vi "Fetch (Scaled and Reduced Resolution).vi"(0 "VISA resource name":refnum<visa-resource-name>, 1 "Segment Index (0)":i32 format="%.0g", 5 "Measurement Source (1: Channel 1)":i32(ring)=1 items=["Channel 1"=1, "Channel 2"=2, "Channel 3"=3, "Channel 4"=4, "Function 1"=5, "Function 2"=6, "Function 3"=7, "Function 4"=8, "Memory 1"=9, "Memory 2"=10, "Memory 3"=11, "Memory 4"=12], 7 "Waveform Size (0)":i32=1000 caption="Waveform Size (1000)", 9 "Maximum Time (10000ms)":u32=10000, 11 "error in (no error)":errorcluster) -> (4 "VISA resource name out":refnum<visa-resource-name>, 6 "Waveform Information":T1, 8 "Waveform Data":waveform(dbl)(graph), 15 "error out":errorcluster)   [LabVIEW 2013, in "Agilent 90000 Series.lvlib"]
doc: "Fetches a decimated and scaled waveform. If the instrument can perform the decimation before pass it to desktop, a decimated waveform will be read directly from the instrument and returned. Else all waveform points will be read from instrument in chunks and a decimation will be perform in the memory of desktop PC. This VI adopts Min/Max decimating method."
uses:
  Agilent 90000 Series.lvlib
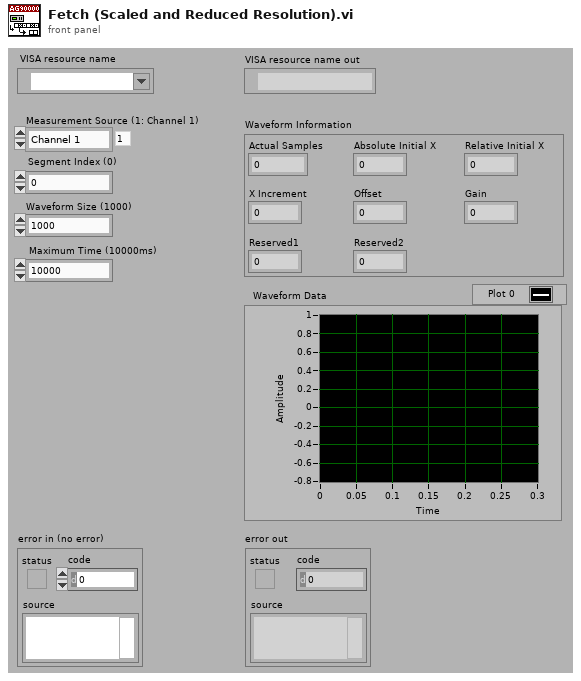
[diagram p1: front panel]
types:
  T1 = cluster{"Actual Samples":i32, "Absolute Initial X":dbl, "Relative Initial X":dbl, "X Increment":dbl, "Offset":dbl, "Gain":dbl, "Reserved1":dbl, "Reserved2":dbl}
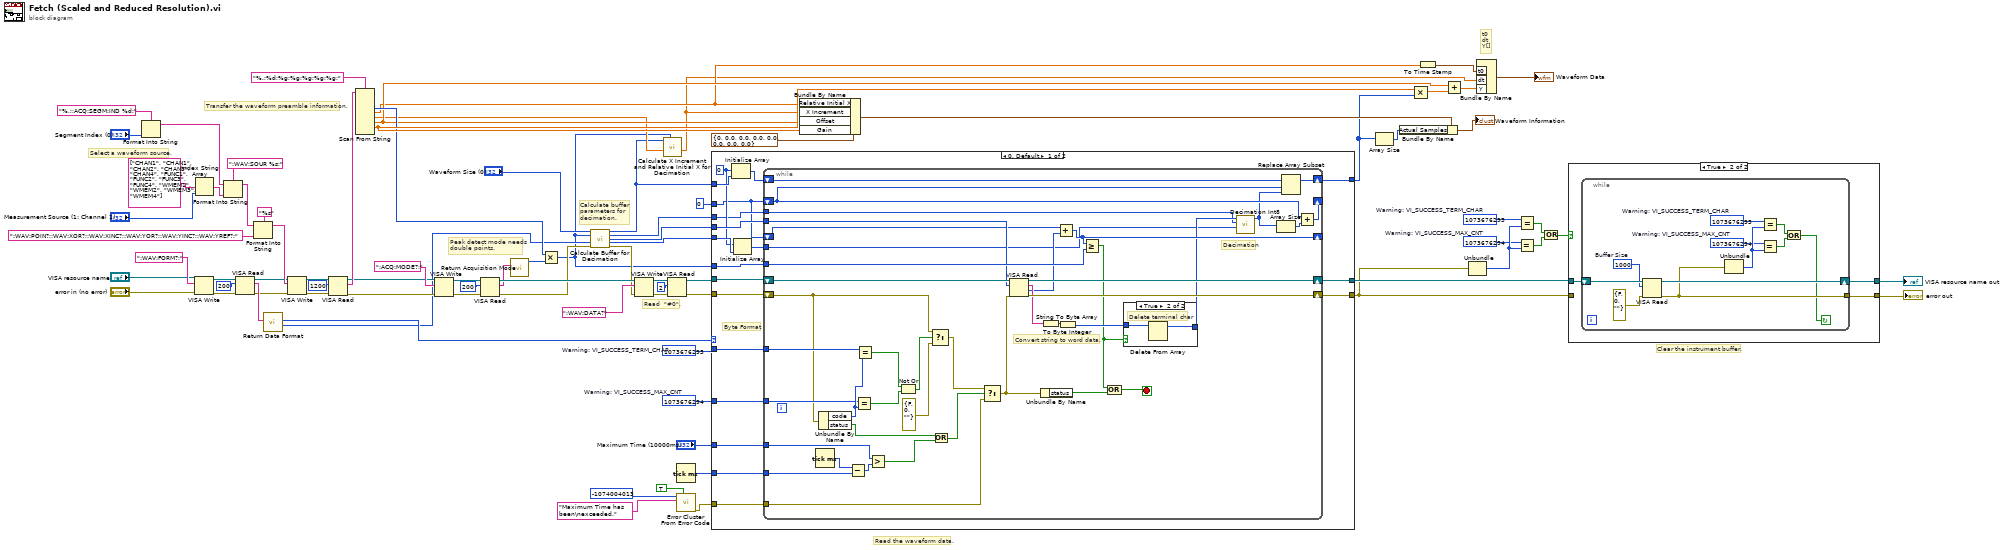
[diagram p0: block diagram]
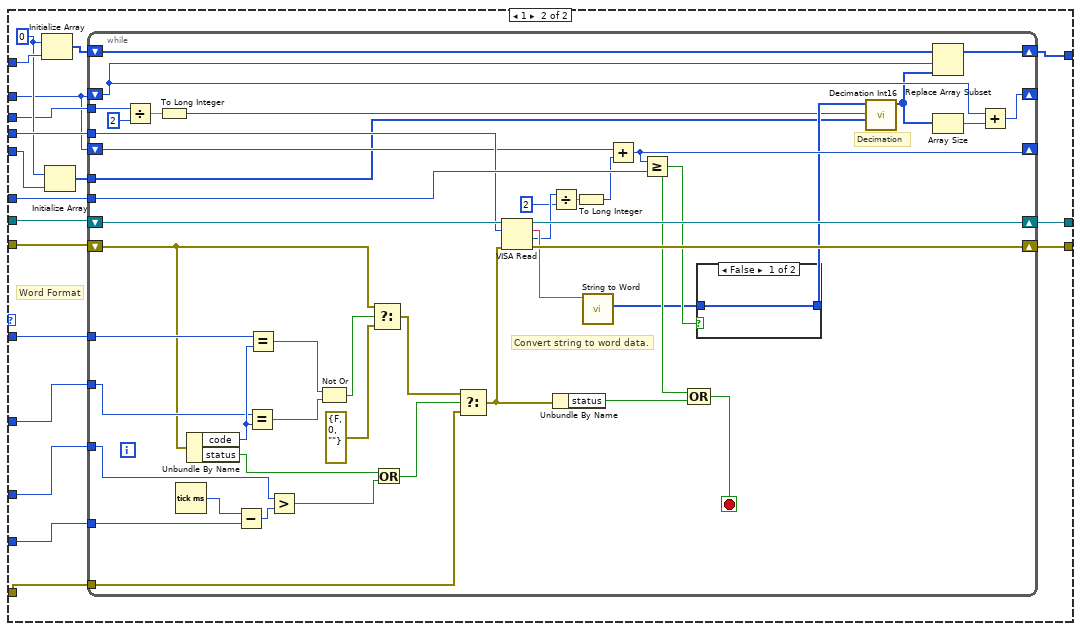
[diagram p3: hidden frame]
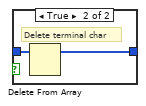
[diagram p4: hidden frame]
diagram:
  w50 = 1073676294  # Warning: VI_SUCCESS_MAX_CNT
  w51 = 1073676293  # Warning: VI_SUCCESS_TERM_CHAR
  w68 = 1073676294  # Warning: VI_SUCCESS_MAX_CNT
  w67 = 1073676293  # Warning: VI_SUCCESS_TERM_CHAR
  # "Calculate buffer \nparameters for \ndecimation."
  # "Read the waveform data."
  # "Peak detect mode needs\ndouble points."
  # "Read  \"#0\"."
  # "Select a waveform source."
  # "t0\ndt\nY[]"
  # "Clear the instrument buffer."
  # "Transfer the waveform preamble information."
  n1 = Format Into String(format string="%.;:ACQ:SEGM:IND %d;", "Segment Index (0)") -> (resulting string=w1:string)  [unwired: 2 in, 1 out]
  n2 = VISA Write(VISA resource name="VISA resource name", write buffer=":WAV:FORM?;", error in (no error)="error in (no error)") -> (VISA resource name out=w43:refnum<visa-resource-name>, error out=w42:errorcluster)  [unwired: 1 out]
  n3 = Index String Array(1:"Measurement Source (1: Channel 1)", 2:string[] ["CHAN1", "CHAN1", "CHAN2", "CHAN3", "CHAN4", "FUNC1", "FUNC2", "FUNC3", "FUNC4", "WMEM1", "WMEM2", "WMEM3", "WMEM4"] ("subarray 2")) -> (0:w76:string)  [unwired: 1 out]
  n4 = Format Into String(format string=":WAV:SOUR %s;" ("Source Command"), initial string=w1, w76) -> (resulting string=w79:string)  [unwired: 1 in, 1 out]
  n5 = VISA Read(VISA resource name=w43, byte count=u32 200, error in (no error)=w42) -> (VISA resource name out=w37:refnum<visa-resource-name>, read buffer=w34:string, error out=w11:errorcluster)  [unwired: 1 out]
  n6 = Format Into String(format string="%s", initial string=w79, ":WAV:POIN?;:WAV:XOR?;:WAV:XINC?;:WAV:YOR?;:WAV:YINC?;:WAV:YREF?;") -> (resulting string=w78:string)  [unwired: 1 in, 1 out]
  n7 = call "Return Data Format.vi"("String In"=w34) -> ("Bytes of Each Point"=w8:u8, "Data Format"=w25:u16)  [unwired: 1 in, 8 out]
  n8 = VISA Write(VISA resource name=w37, write buffer=w78, error in (no error)=w11) -> (VISA resource name out=w84:refnum<visa-resource-name>, error out=w83:errorcluster)  [unwired: 1 out]
  n9 = VISA Read(VISA resource name=w84, byte count=u32 1200, error in (no error)=w83) -> (VISA resource name out=w32:refnum<visa-resource-name>, read buffer=w62:string, error out=w12:errorcluster)  [unwired: 1 out]
  n10 = Scan From String(format string="%.;%d;%g;%g;%g;%g;%g;", input string=w62) -> (output 1=w28:i32, output 2=w13:dbl, output 3=w10:dbl, output 4=w14:dbl, output 5=w29:dbl)  [unwired: 2 in, 10 out]
  n11 = VISA Write(VISA resource name=w32, write buffer=":ACQ:MODE?;", error in (no error)=w12) -> (VISA resource name out=w58:refnum<visa-resource-name>, error out=w59:errorcluster)  [unwired: 1 out]
  n12 = VISA Read(VISA resource name=w58, byte count=u32 200, error in (no error)=w59) -> (VISA resource name out=w57:refnum<visa-resource-name>, read buffer=w15:string, error out=w18:errorcluster)  [unwired: 1 out]
  n13 = call "Return Acquisition Mode.vi"("Acquisition Mode"=w15) -> ("Multiply Factor"=w16:i32)  [unwired: 10 out]
  n14 = Multiply(x=w28, y=w16) -> (x*y=w6:i32)
  n15 = call "Calculate Buffer for Decimation.vi"("Waveform Size In (100)"="Waveform Size (0)", "Actual Points (1000)"=w6, "Bytes of Each Point (1)"=w8, "error in (no error)"=w18) -> ("Waveform Size Out"=w4:i32, "Number of Bytes per Chunck"=w5:i32, "Number of Bytes per Fetch"=w20:i32, "Decimation Buffer Size"=w19:i32, "error out"=w17:errorcluster)  [unwired: 7 out]
  n16 = VISA Write(VISA resource name=w57, write buffer=":WAV:DATA?" ("format string"), error in (no error)=w17) -> (VISA resource name out=w65:refnum<visa-resource-name>, error out=w64:errorcluster)  [unwired: 1 out]
  n17 = call "Calculate X Increment and Relative Initial X for Decimation.vi"("Actual Points (1000)"=w6, "Original X Increment (0)"=w10, "Waveform Size (100)"=w4) -> ("X Increment Out"=w9:dbl)  [unwired: 2 in, 6 out]
  n18 = VISA Read(VISA resource name=w65, byte count=u32 2, error in (no error)=w64) -> (VISA resource name out=w35:refnum<visa-resource-name>, error out=w36:errorcluster)  [unwired: 2 out]
  n19 = Tick Count (ms)() -> (millisecond timer value=w48:u32)
  n20 = call <vilib>:"Error Cluster From Error Code.vi"("show call chain? (False)"=TRUE, "error message (\"\")"="Maximum Time has been\nexceeded." ("error message (\"\")"), "error code (0)"=-1074004013) -> ("error out"=w45:errorcluster)  [unwired: 1 in, 5 out]
  n21 = case shown="0, Default" w25 {
    tunnel: [w103 w166] -> w74
    tunnel: [w102 w165] -> w73
    tunnel: w36 -> [w101 w164]
    tunnel: w35 -> [w100 w163]
    tunnel: [w99 w162] -> w23
    tunnel: w51 -> [w98 w161]
    tunnel: w50 -> [w97 w160]
    tunnel: "Maximum Time (10000ms)" -> [w96 w159]
    tunnel: w48 -> [w95 w158]
    tunnel: w45 -> [w94 w157]
    tunnel: w4 -> [w92 w155]
    tunnel: w20 -> [w91 w154]
    tunnel: w6 -> [w90 w153]
    tunnel: w19 -> [w89 w152]
    tunnel: w5 -> [w86 w149]
    tunnel: 0 ("index") -> [w85 w148]
    frame 0, Default {
      w88 = i8 0 ("element")
      # "Byte Format"
      n22 = Initialize Array(w88, w92) -> (w93:i8[])
      n23 = Initialize Array(w88, w89) -> (w87:i8[])
      n24 = while {
        shift-right: [w141] -> w102
        shift-left: w101 -> [w132]
        shift-right: [w144] -> w103
        shift-left: w100 -> [w143]
        shift-right: [w142] -> w99
        shift-left: w93 -> [w119]
        shift-right: [w140] -> _
        shift-left: w85 -> [w112]
        tunnel: w98 -> [w134]
        tunnel: w97 -> [w133]
        tunnel: w96 -> [w129]
        tunnel: w95 -> [w128]
        tunnel: w94 -> [w123]
        tunnel: w90 -> [w116]
        tunnel: w91 -> [w115]
        tunnel: w86 -> [w106]
        tunnel: w87 -> [w105]
        shift-right: [w110] -> _
        shift-left: w85 -> [w108]
        stop <- w120 stop-if-true
        # "Convert string to word data."
        # "Decimation"
        n25 = Tick Count (ms)() -> (millisecond timer value=w130:u32)
        n26 = Unbundle By Name(w132) -> ("code"=w135:i32, "status"=w127:bool)
        n27 = Subtract(x=w130, y=w128) -> (x-y=w131:u32)
        n28 = Equal?(x=w133, y=w135) -> (x = y?=w138:bool)
        n29 = Equal?(x=w134, y=w135) -> (x = y?=w139:bool)
        n30 = Greater?(x=w129, y=w131) -> (0:w126:bool)
        n31 = Not Or(1:w138, 2:w139) -> (0:w137:bool)
        n32 = Select(t=w132, s=w137, f=errorcluster {"status"=FALSE, "code"=0, "source"=""} ("error in (no error)")) -> (s? t:f=w125:errorcluster)
        n33 = Or(x=w127, y=w126) -> (x .or. y?=w124:bool)
        n34 = Select(t=w125, s=w124, f=w123) -> (s? t:f=w122:errorcluster)
        n35 = VISA Read(VISA resource name=w143, byte count=w115, error in (no error)=w122) -> (VISA resource name out=w144:refnum<visa-resource-name>, read buffer=w118:string, return count=w114:u32, error out=w141:errorcluster)
        n36 = Unbundle By Name(w122) -> ("status"=w121:bool)
        n37 = String To Byte Array(string=w118) -> (unsigned byte array=w117:u8[])
        n38 = Add(x=w112, y=w114) -> (x+y=w140:u32)
        n39 = To Byte Integer(number=w117) -> (8bit integer=w113:i8[])
        n40 = Greater Or Equal?(x=w140, y=w116) -> (x >= y?=w109:bool)
        n41 = Compound Arithmetic op=OR(w109, w121) -> (w120:bool)
        n42 = case shown="True" w109 {
          tunnel: w113 -> [w145 w147]
          tunnel: [w145 w146] -> w107
          frame False {
          }
          frame True {
            # "Delete terminal char"
            n43 = Delete From Array(array=w147) -> (array with subset deleted=w146:i8[])  [unwired: 2 in, 1 out]
          }
        }
        n44 = call "Decimation Int8.vi"("Decimation Array"=w105, "Number of Bytes per Chunck (1000)"=w106, "Raw Data"=w107) -> ("Decimation Data"=w104:i8[])  [unwired: 8 out]
        n45 = Array Size(array=w104) -> (size(s)=w111:i32)
        n46 = Replace Array Subset(array=w119, new element=w104, index=w108) -> (w142:i8[])
        n47 = Add(x=w108, y=w111) -> (x+y=w110:i32)
      }
    }
    frame 1 {
      w151 = i16 0 ("element")
      # "Word Format"
      n48 = Initialize Array(w151, w155) -> (w156:i16[])
      n49 = Initialize Array(w151, w152) -> (w150:i16[])
      n50 = while {
        shift-right: [w209] -> w165
        shift-left: w164 -> [w200]
        shift-right: [w212] -> w166
        shift-left: w163 -> [w211]
        shift-right: [w210] -> w162
        shift-left: w156 -> [w187]
        shift-right: [w208] -> _
        shift-left: w148 -> [w184]
        tunnel: w161 -> [w202]
        tunnel: w160 -> [w201]
        tunnel: w159 -> [w197]
        tunnel: w158 -> [w196]
        tunnel: w157 -> [w191]
        tunnel: w153 -> [w186]
        tunnel: w154 -> [w185]
        tunnel: w149 -> [w173]
        tunnel: w150 -> [w167]
        shift-right: [w181] -> _
        shift-left: w148 -> [w183]
        stop <- w188 stop-if-true
        # "Decimation"
        # "Convert string to word data."
        n51 = Divide(x=w173, y=2) -> (x/y=w172:dbl)
        n52 = To Long Integer(number=w172) -> (32bit integer=w168:i32)
        n53 = Tick Count (ms)() -> (millisecond timer value=w198:u32)
        n54 = Unbundle By Name(w200) -> ("code"=w203:i32, "status"=w195:bool)
        n55 = Subtract(x=w198, y=w196) -> (x-y=w199:u32)
        n56 = Equal?(x=w201, y=w203) -> (x = y?=w206:bool)
        n57 = Equal?(x=w202, y=w203) -> (x = y?=w207:bool)
        n58 = Greater?(x=w197, y=w199) -> (0:w194:bool)
        n59 = Not Or(1:w206, 2:w207) -> (0:w205:bool)
        n60 = Select(t=w200, s=w205, f=errorcluster {"status"=FALSE, "code"=0, "source"=""} ("error in (no error)")) -> (s? t:f=w193:errorcluster)
        n61 = Or(x=w195, y=w194) -> (x .or. y?=w192:bool)
        n62 = Select(t=w193, s=w192, f=w191) -> (s? t:f=w190:errorcluster)
        n63 = VISA Read(VISA resource name=w211, byte count=w185, error in (no error)=w190) -> (VISA resource name out=w212:refnum<visa-resource-name>, read buffer=w179:string, return count=w176:u32, error out=w209:errorcluster)
        n64 = Divide(x=w176, y=u32 2) -> (x/y=w177:dbl)
        n65 = Unbundle By Name(w190) -> ("status"=w189:bool)
        n66 = To Long Integer(number=w177) -> (32bit integer=w175:i32)
        n67 = call "String to Word.vi"("String"=w179) -> ("Int16 Data"=w178:i16[])  [unwired: 1 in, 9 out]
        n68 = Add(x=w184, y=w175) -> (x+y=w208:i32)
        n69 = Greater Or Equal?(x=w208, y=w186) -> (x >= y?=w180:bool)
        n70 = Compound Arithmetic op=OR(w180, w189) -> (w188:bool)
        n71 = case shown="False" w180 {
          tunnel: w178 -> [w213 w215]
          tunnel: [w213 w214] -> w169
          frame False {
          }
          frame True {
            # "Delete terminal char"
            n72 = Delete From Array(array=w215) -> (array with subset deleted=w214:i16[])  [unwired: 2 in, 1 out]
          }
        }
        n73 = call "Decimation Int16.vi"("Decimation Array"=w167, "Number of Bytes per Chunck (1000)"=w168, "Raw Data"=w169) -> ("Decimation Data"=w170:i16[])  [unwired: 8 out]
        n74 = Replace Array Subset(array=w187, new element=w170, index=w183) -> (w210:i16[])
        n75 = Array Size(array=w170) -> (size(s)=w182:i32)
        n76 = Add(x=w183, y=w182) -> (x+y=w181:i32)
      }
    }
  }
  n77 = Bundle By Name(cluster=T1 {"Actual Samples"=0, "Absolute Initial X"=0.0, "Relative Initial X"=0.0, "X Increment"=0.0, "Offset"=0.0, "Gain"=0.0, "Reserved1"=0.0, "Reserved2"=0.0} ("Waveform Information"), "Relative Initial X"=w13, "X Increment"=w9, "Offset"=w14, "Gain"=w29) -> (w60:T1)
  n78 = Array Size(array=w23) -> (size(s)=w21:i32)
  n79 = Bundle By Name(cluster=w60, "Actual Samples"=w21) -> (→"Waveform Information":T1)
  n80 = Multiply(x=w29, y=w23) -> (x*y=w53:dbl[])
  n81 = To Time Stamp(1:w13) -> (0:w56:timestamp)
  n82 = Add(x=w14, y=w53) -> (x+y=w54:dbl[])
  n83 = Unbundle(w73) -> ("code"=w69:i32)  [unwired: 2 out]
  n84 = Bundle By Name ("Build Waveform")("t0"=w56, "dt"=w9, "Y"=w54) -> (→"Waveform Data":waveform(dbl))  [unwired: 1 out]
  n85 = Equal?(x=w68, y=w69) -> (x = y?=w71:bool)
  n86 = Equal?(x=w67, y=w69) -> (x = y?=w72:bool)
  n87 = Or(x=w72, y=w71) -> (x .or. y?=w70:bool)
  n88 = case shown="True" w70 {
    tunnel: w74 -> [w217 w220]
    tunnel: w73 -> [w216 _]
    tunnel: [w217 w219] -> w31
    tunnel: [w216 w218] -> w30
    frame False {
    }
    frame True {
      n89 = while {
        shift-right: [w230] -> w219
        shift-left: w220 -> [w231]
        tunnel: [w223] -> w218
        stop <- w222 continue-if-true
        w225 = 1073676294  # Warning: VI_SUCCESS_MAX_CNT
        w224 = 1073676293  # Warning: VI_SUCCESS_TERM_CHAR
        w229 = u32 1000  # Buffer Size
        n90 = VISA Read(VISA resource name=w231, byte count=w229, error in (no error)=errorcluster {"status"=FALSE, "code"=0, "source"=""}) -> (VISA resource name out=w230:refnum<visa-resource-name>, error out=w223:errorcluster)  [unwired: 2 out]
        n91 = Unbundle(w223) -> ("code"=w226:i32)  [unwired: 2 out]
        n92 = Equal?(x=w225, y=w226) -> (x = y?=w227:bool)
        n93 = Equal?(x=w224, y=w226) -> (x = y?=w228:bool)
        n94 = Or(x=w228, y=w227) -> (x .or. y?=w222:bool)
      }
    }
  }
  "error out" <- w30
  "VISA resource name out" <- w31
